vi "Format Site List.vi"(7 "Bus Number":i32) -> (8 "Site List":string)   [LabVIEW 2018, in "MIPI RFFE API.lvlib"]
uses:
  MIPI RFFE API.lvlib
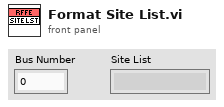
[diagram p1: front panel]
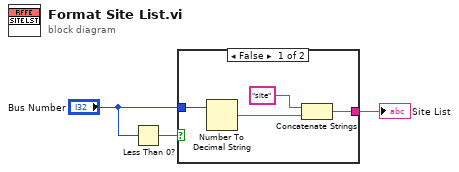
[diagram p0: block diagram]
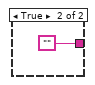
[diagram p2: hidden frame]
diagram:
  n1 = Less Than 0?(x="Bus Number") -> (x < 0?=w1:bool)
  n2 = case shown="False" w1 {
    tunnel: [w5 ""] -> w3
    tunnel: "Bus Number" -> [w4 _]
    frame False {
      n3 = Number To Decimal String(number=w4) -> (decimal integer string=w7:string)  [unwired: 1 in]
      n4 = Concatenate Strings("site" ("string"), w7) -> (w5:string)
    }
    frame True {
    }
  }
  "Site List" <- w3
